vi "Calculate Path.vi"(8 "error in (no error)":errorcluster, 10 "Direction Heading":T1, 11 "Module Data in":refnum<class "Grassfire Algorithm.lvclass">) -> (0 "error out":errorcluster, 1 "Directions":T1[](array[typedef]), 2 "Solution":T2[][](array[typedef]), 3 "Module Data out":refnum<class "Grassfire Algorithm.lvclass">)   [LabVIEW 2019, in "Grassfire Algorithm.lvclass"]
uses:
  Grassfire Algorithm.lvclass
  Solution Grid Cell--cluster.ctl
  Solution--picture ring.ctl
  Direction--enum.ctl
  Grassfire Algorithm.lvclass/Grassfire Algorithm.ctl
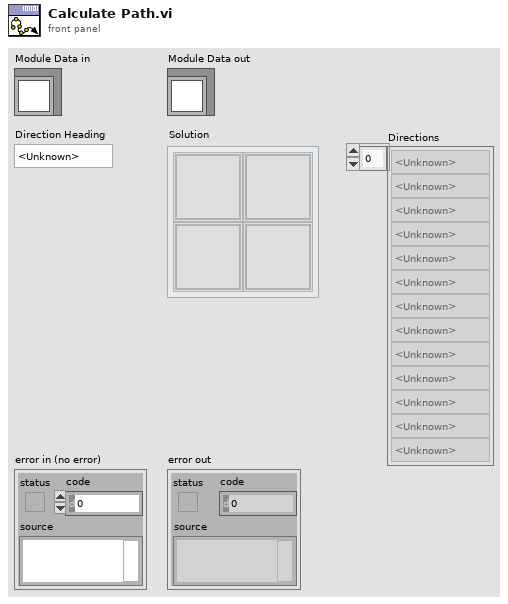
[diagram p1: front panel]
types:
  T1 = typedef "Grassfire Algorithm.lvclass/Direction--enum.ctl" = enum16{"<Unknown>", "Right", "Down", "Left", "Up"}
  T2 = typedef "Grassfire Algorithm.lvclass/Solution Grid Cell--cluster.ctl" = cluster{"Picture":T3, "Value":string}
  T3 = typedef "Grassfire Algorithm.lvclass/Solution--picture ring.ctl" = i64
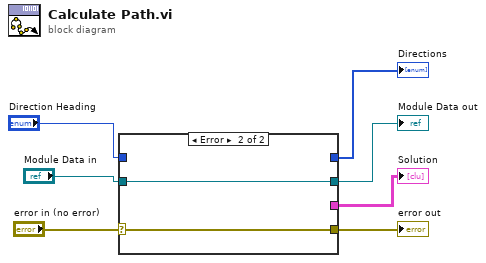
[diagram p0: block diagram]
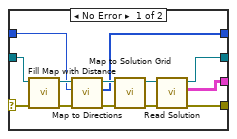
[diagram p2: hidden frame]
diagram:
  n1 = case shown="Error" "error in (no error)" {
    selector: "error in (no error)" -> [w19 w22]
    tunnel: [w17 w22] -> w6
    tunnel: [w18 w21] -> w4
    tunnel: "Module Data in" -> [w20 w21]
    tunnel: [w16 _] -> w3
    tunnel: "Direction Heading" -> [w9 _]
    tunnel: [w8 _] -> w1
    frame No Error {
      n2 = call "Fill Map with Distance.vi"("error in (no error)"=w19, "Grassfire Algorithm in"=w20) -> ("error out"=w14:errorcluster, "Grassfire Algorithm out"=w15:refnum<class "Grassfire Algorithm.lvclass">)  [unwired: 8 in]
      n3 = call "Map to Directions.vi"("error in (no error)"=w14, "Direction Heading"=w9, "Grassfire Algorithm in"=w15) -> ("error out"=w12:errorcluster, "Directions"=w8:T1[], "Grassfire Algorithm out"=w13:refnum<class "Grassfire Algorithm.lvclass">)  [unwired: 6 in]
      n4 = call "Map to Solution Grid.vi"("error in (no error)"=w12, "Grassfire Algorithm in"=w13) -> ("error out"=w10:errorcluster, "Grassfire Algorithm out"=w11:refnum<class "Grassfire Algorithm.lvclass">)  [unwired: 8 in]
      n5 = call "Read Solution.vi"("error in (no error)"=w10, "Module Data in"=w11) -> ("error out"=w17:errorcluster, "Solution"=w16:T2[][], "Module Data out"=w18:refnum<class "Grassfire Algorithm.lvclass">)  [unwired: 7 in]
    }
    frame Error {
    }
  }
  "error out" <- w6
  "Module Data out" <- w4
  "Solution" <- w3
  "Directions" <- w1
